vi "SubVI Tester.vi"() -> ()   [LabVIEW 2015]
panel:
  in  "WeatherData":T1={"Current Temperature"=0.0, "Max Temperature"=0.0, "Min Temperature"=0.0, "Warning Text"="No Warning", "Warning?"=FALSE}
  out "WeatherData OUT 2":T1={"Current Temperature"=0.0, "Max Temperature"=0.0, "Min Temperature"=0.0, "Warning Text"="No Warning", "Warning?"=FALSE}
  in  "Min Temperature":dbl=10.0
  in  "Max Temperature":dbl=30.0
  in  "Stop":bool
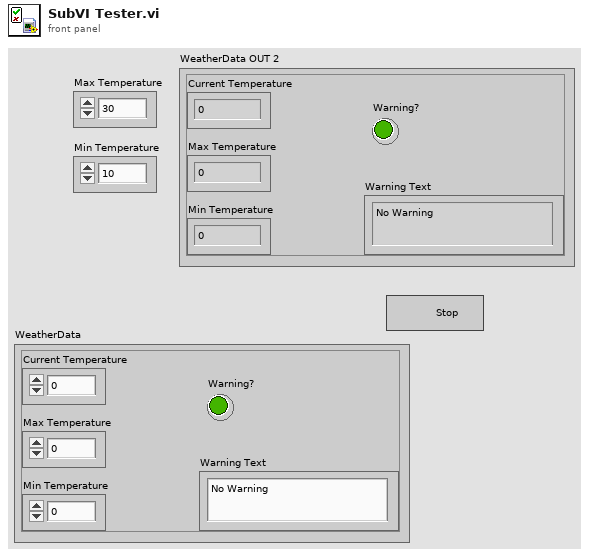
[diagram p1: front panel]
types:
  T1 = cluster{"Current Temperature":dbl, "Max Temperature":dbl, "Min Temperature":dbl, "Warning Text":string, "Warning?":bool}
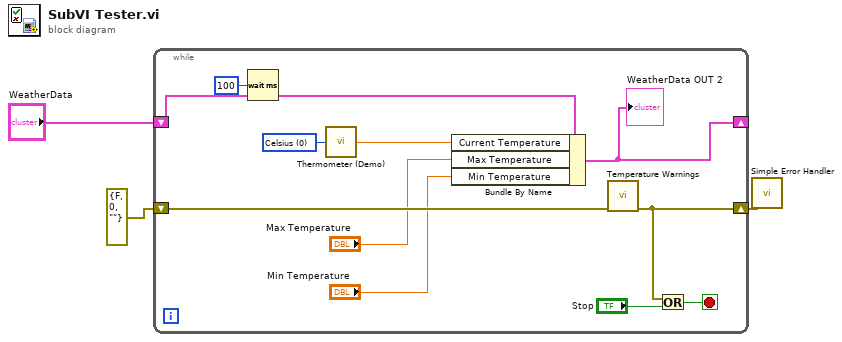
[diagram p0: block diagram]
diagram:
  n1 = while {
    shift-right: [w10] -> w3
    shift-left: errorcluster {"status"=FALSE, "code"=0, "source"=""} ("error out") -> [w11]
    shift-right: [w4] -> _
    shift-left: "WeatherData" -> [w8]
    stop <- w12 stop-if-true
    w9 = u16 0 items=["Celsius", "Fahrenheit"] ("Units (0: Celsius)")
    n2 = Wait (ms)(milliseconds to wait=u32 100) -> ()  [unwired: 1 out]
    n3 = call "Thermometer (Demo).vi"("Units (0: Celsius)"=w9) -> ("Temperature Value"=w7:dbl)
    n4 = Bundle By Name(cluster=w8, "Current Temperature"=w7, "Max Temperature"="Max Temperature", "Min Temperature"="Min Temperature") -> (w4:T1)
    "WeatherData OUT 2" <- w4
    n5 = call "Temperature Warnings.vi"("Error In"=w11) -> ("Error Out"=w10:errorcluster)  [unwired: 9 in, 1 out]
    n6 = Or(x=w10, y="Stop") -> (x .or. y?=w12:bool)
  }
  n7 = call <vilib>:"Simple Error Handler.vi"("error in (no error)"=w3) -> ()  [unwired: 4 in, 5 out]
